vi "AxisControl.vi"(0 "String in":string, 1 "AxisBounds":T5={"Min"={"Auto"=TRUE, "Value"=0.0}, "Max"={"Auto"=TRUE, "Value"=0.0}}, 2 "Time Format String":string, 3 "ticsAndGrids":T2={"tics"={"ticMin"=0.0, "ticStep"=0.0, "ticMax"=0.0, "minorDivsPerMajor"=2, "ticSpacing"=enum."Auto Tics", "ticPosition"=enum."Inside, no mirror"}, "Grids"={"Gridlines"=enum."Major grid", "Zeroaxis"=enum."No zero axis"}, "Mapping"=enum."Lin"}, 5 "Axis":T7="x", 7 "Time format?":bool, 9 "ShowNumbers?":bool=TRUE, 11 "ShowLabel?":bool=TRUE, 12 "Axis Label":string, 13 "DataSpan":cluster{"Max":dbl, "Min":dbl}, 14 "AdditionalTics":dbl[](array[numeric])) -> (4 "String out":string, 6 "Commands":T1)   [LabVIEW 2022 SP3]
uses:
  axisName.ctl
  minAndMax.ctl
  AutoManualNumber.ctl
  ticsAndGrids.ctl
  tics.ctl
  grids.ctl
  commandArray.ctl
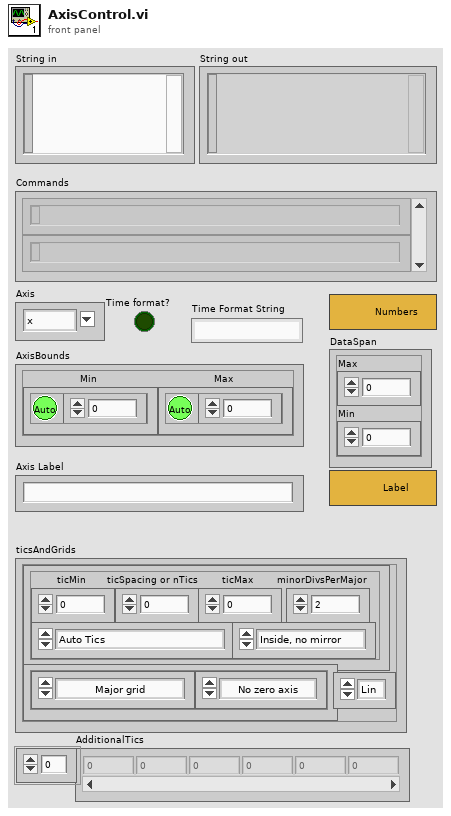
[diagram p1: front panel]
types:
  T1 = typedef "commandArray.ctl" = string[]
  T2 = typedef "ticsAndGrids.ctl" = cluster{"tics":T3, "Grids":T4, "Mapping":enum8{"Lin", "Log"}}
  T3 = typedef "tics.ctl" = cluster{"ticMin":dbl, "ticStep":dbl, "ticMax":dbl, "minorDivsPerMajor":i32, "ticSpacing":enum16{"Auto Tics", "Fixed spacing", "Fixed Minimum and Spacing", "Start, Spacing and Maximum", "Approx n Tics (rounded)"}, "ticPosition":enum16{"Inside, no mirror", "Inside, mirrored", "Outside, no mirror", "Outside, mirrored", "Invisible"}}
  T4 = typedef "grids.ctl" = cluster{"Gridlines":enum16{"No grids", "Major grid", "Minor grid", "Major and Minor"}, "Zeroaxis":enum16{"No zero axis", "Show zero axis"}}
  T5 = typedef "minAndMax.ctl" = cluster{"Min":T6, "Max":T6}
  T6 = typedef "AutoManualNumber.ctl" = cluster{"Auto":bool, "Value":dbl}
  T7 = typedef "axisName.ctl" = string
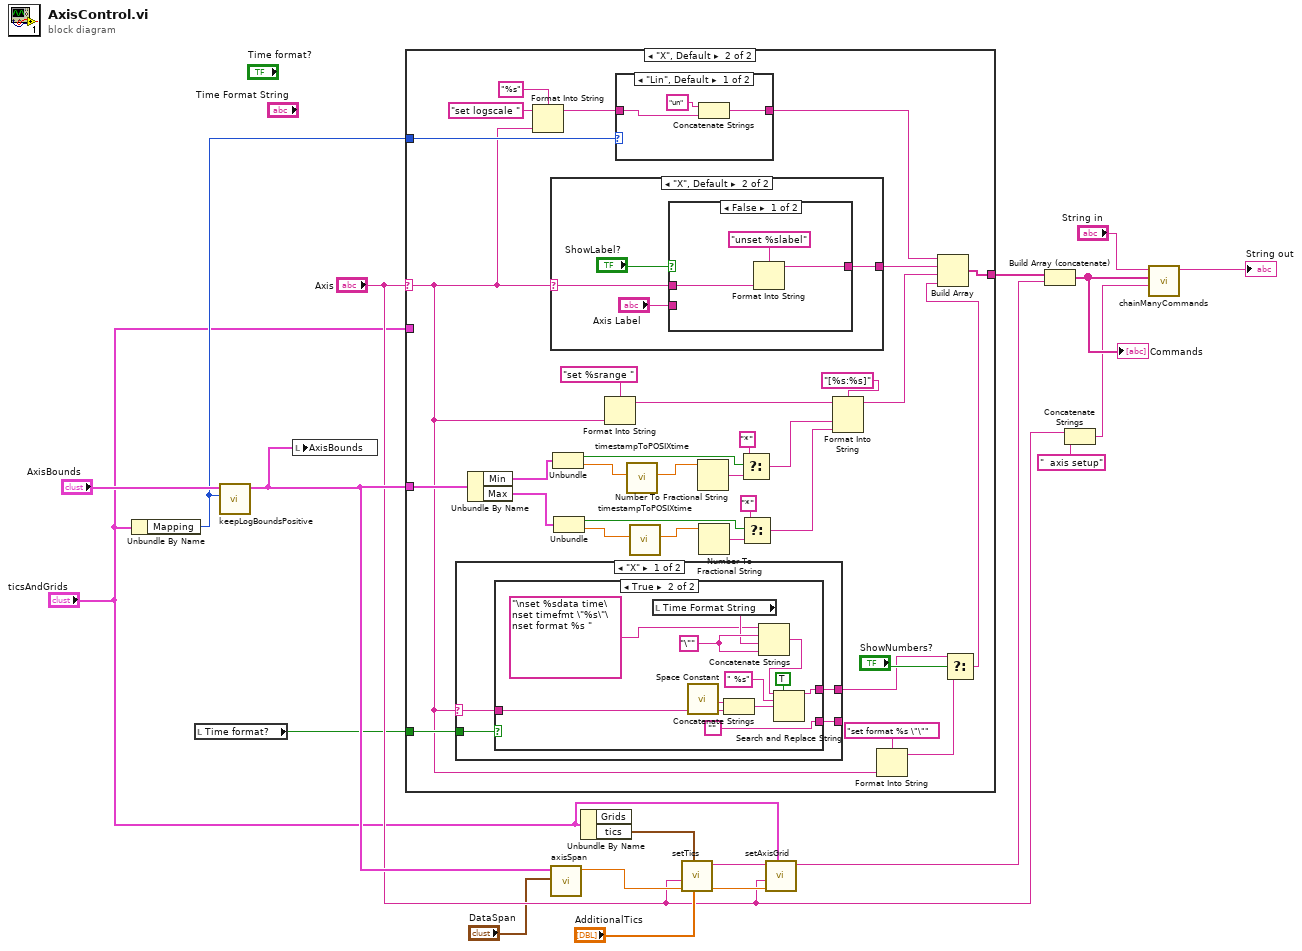
[diagram p0: block diagram]
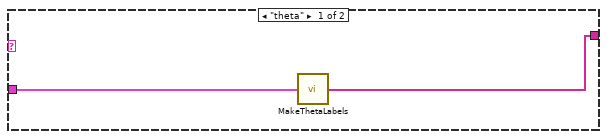
[diagram p2: hidden frame]
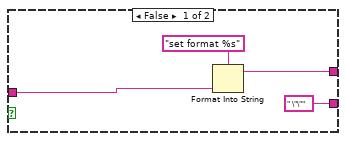
[diagram p3: hidden frame]
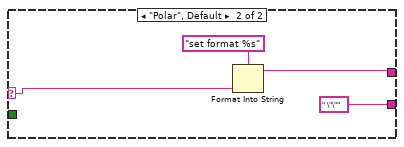
[diagram p4: hidden frame]
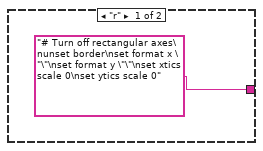
[diagram p6: hidden frame]
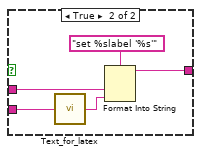
[diagram p7: hidden frame]
diagram:
  n1 = Unbundle By Name("ticsAndGrids") -> ("Mapping"=w4:enum8{"Lin", "Log"})
  n2 = local read "Time format?"() -> (w1:bool)
  n3 = call "keepLogBoundsPositive.vi"("Mapping"=w4, "AxisBounds in"="AxisBounds") -> ("AxisBounds out"=w9:T5)  [unwired: 9 in]
  n4 = local write "AxisBounds"(w9) -> ()
  n5 = case shown="\"X\", Default" "Axis" {
    selector: "Axis" -> [_ w23]
    tunnel: [w20 w50] -> w17
    tunnel: w9 -> [_ w36]
    tunnel: w4 -> [_ w35]
    tunnel: "ticsAndGrids" -> [w21 _]
    tunnel: w1 -> [_ w25]
    frame "theta" {
      n6 = call "MakeThetaLabels.vi"("ticsAndGrids"=w21) -> ("Theta Label Command String"=w20:string[])
    }
    frame "X", Default {
      n7 = case shown="\"X\"" w23 {
        selector: w23 -> [w57 w76]
        tunnel: [w58 w75] -> w30
        tunnel: [w56 " \"\"" ("format string")] -> _
        tunnel: w25 -> [w55 _]
        frame "X" {
          n8 = case shown="True" w55 {
            tunnel: [w61 w69] -> w58
            tunnel: w57 -> [w60 w68]
            tunnel: [" \"\"" ("format string") ""] -> w56
            frame False {
              n9 = Format Into String(format string="set format %s", w60) -> (resulting string=w61:string)  [unwired: 2 in, 1 out]
            }
            frame True {
              w67 = "\""
              n10 = local read "Time Format String"() -> (w66:string)
              n11 = call <vilib>:"Space Constant.vi"() -> ("String"=w72:string)
              n12 = Concatenate Strings(w72, w68) -> (w73:string)
              n13 = Concatenate Strings("\nset %sdata time\nset timefmt \"%s\"\nset format %s ", w67, w66, w67) -> (w64:string)
              n14 = Search and Replace String(replace all?=TRUE ("replace all? (F)"), input string=w64, search string=" %s", replace string=w73) -> (result string=w69:string)  [unwired: 4 in, 3 out]
            }
          }
        }
        frame "Polar", Default {
          n15 = Format Into String(format string="set format %s", w76) -> (resulting string=w75:string)  [unwired: 2 in, 1 out]
        }
      }
      n16 = Unbundle By Name(w36) -> ("Min"=w38:T6, "Max"=w37:T6)
      n17 = Format Into String(format string="%s", initial string="set logscale ", w23) -> (resulting string=w32:string)  [unwired: 1 in, 1 out]
      n18 = case shown="\"X\", Default" w23 {
        selector: w23 -> [_ w84]
        tunnel: ["# Turn off rectangular axes\nunset border\nset format x \"\"\nset format y \"\"\nset xtics scale 0\nset ytics scale 0" w85] -> w48
        frame "r" {
        }
        frame "X", Default {
          n19 = case shown="False" "ShowLabel?" {
            tunnel: w84 -> [w88 w93]
            tunnel: [w87 w92] -> w85
            tunnel: "Axis Label" -> [_ w90]
            frame False {
              n20 = Format Into String(format string="unset %slabel", w88) -> (resulting string=w87:string)  [unwired: 2 in, 1 out]
            }
            frame True {
              n21 = call "Text_for_latex.vi"("Input String"=w90) -> ("Output String"=w91:string)
              n22 = Format Into String(format string="set %slabel '%s'", w93, w91) -> (resulting string=w92:string)  [unwired: 2 in, 1 out]
            }
          }
        }
      }
      n23 = Unbundle(w38) -> ("Auto"=w44:bool, "Value"=w29:dbl)
      n24 = Unbundle(w37) -> ("Auto"=w42:bool, "Value"=w27:dbl)
      n25 = Format Into String(format string="set %srange ", w23) -> (resulting string=w53:string)  [unwired: 2 in, 1 out]
      n26 = case shown="\"Lin\", Default" w35 {
        tunnel: [w79 w81] -> w31
        tunnel: w32 -> [w80 w81]
        frame "Lin", Default {
          n27 = Concatenate Strings("un" ("string"), w80) -> (w79:string)
        }
        frame "Log" {
        }
      }
      n28 = call "timestampToPOSIXtime.vi"("numberToTest"=w29) -> ("numberOut"=w28:dbl)  [unwired: 8 in, 2 out]
      n29 = call "timestampToPOSIXtime.vi"("numberToTest"=w27) -> ("numberOut"=w26:dbl)  [unwired: 8 in, 2 out]
      n30 = Number To Fractional String(number=w28) -> (F-format string=w46:string)  [unwired: 3 in]
      n31 = Number To Fractional String(number=w26) -> (F-format string=w40:string)  [unwired: 3 in]
      n32 = Select(t="*", s=w44, f=w46) -> (s? t:f=w43:string)
      n33 = Select(t="*", s=w42, f=w40) -> (s? t:f=w39:string)
      n34 = Format Into String(format string="[%s:%s]", initial string=w53, w43, w39) -> (resulting string=w52:string)  [unwired: 1 in, 1 out]
      n35 = Format Into String(format string="set format %s \"\"", w23) -> (resulting string=w22:string)  [unwired: 2 in, 1 out]
      n36 = Select(t=w30, s="ShowNumbers?", f=w22) -> (s? t:f=w49:string)
      n37 = Build Array(w31, w48, w52, w49) -> (w50:string[])
    }
  }
  n38 = call "axisSpan.vi"("DataSpan"="DataSpan", "AxisBounds"=w9) -> ("ActualSpan"=w11:dbl)  [unwired: 9 in]
  n39 = Unbundle By Name("ticsAndGrids") -> ("tics"=w18:T3)  [unwired: 1 out]
  n40 = call "setTics.vi"("AdditionalTics"="AdditionalTics", "tics"=w18, "AxisSpan"=w11, "Axis"="Axis") -> ("polarGrid"=w15:dbl, "String out"=w19:string)  [unwired: 6 in]
  n41 = call "setAxisGrid.vi"("ticsAndGrids"="ticsAndGrids", "polarGridAngle"=w15, "Axis"="Axis", "String in"=w19) -> ("String out"=w16:string)  [unwired: 7 in]
  n42 = Build Array (concatenate)(w17, w16) -> (w12:string[])
  "Commands" <- w12
  n43 = Concatenate Strings("Axis", "  axis setup" ("string")) -> (w7:string)
  n44 = call "chainManyCommands.vi"("Comments"=w7, "CommandArray"=w12, "String in in"="String in") -> ("String out"=→"String out":string)  [unwired: 8 in]
